vi "hind brain 3.vi"() -> ()   [LabVIEW 2011, in "Hindbrain Demo.lvrbt"]
uses:
  Hindbrain Demo.lvrbt
  <vilib>/NXT/Block Support/HWPage.SensorType.ctl
  <vilib>/NXT/Block Support/HWPage.SensorMode.ctl
  <vilib>/NXT/Block Support/NXT_InputPort.ctl
  <vilib>/NXT/Subs/MotorOutput.ctl
  <vilib>/NXT/HiTechnic/HiTechnic Controls/HiTechnic Port.ctl
  <vilib>/NXT/Dual Mode Library/Motors/MotorBrake.vi
  <vilib>/NXT/Dual Mode Library/Motors/MotorOn.vi
  <vilib>/NXT/Dual Mode Library/Motors/MotorReverse.vi
  New Sensors/mindsensors.com_LVEE_Toolkit/mindsensors.com_LVEE_Toolkit_V1.23/mindsensors.com LVEE Toolkit/Dual/Distance Sensor-DM.vi
  New Sensors/mindsensors.com_LVEE_Toolkit/mindsensors.com_LVEE_Toolkit_V1.23/mindsensors.com LVEE Toolkit/Dual/NXTServo-DM.vi
panel:
  in  "Thrust\nAction":i32
  out "Distance Value":ext
  out "Signal Strength (Array)":u8[](array[numeric])
  out "Direction (0-9)":i16
  in  "Input of NXTServo 2":T1={"Servo Number"=2, "Position"=1500, "Speed"=0} {"Speed" step=1 scale=0.0..255.0; "Position" min=500 max=2500 step=1 scale=500.0..2500.0; "Servo Number" min=1 max=8 step=1}
  out "Output of NXTServo 2":cluster{"Voltage":u8, "Status":bool}
  in  "stop":bool
  in  "Input of NXTServo":T1={"Servo Number"=1, "Position"=1500, "Speed"=0} {"Speed" step=1 scale=0.0..255.0; "Position" min=500 max=2500 step=1 scale=500.0..2500.0; "Servo Number" min=1 max=8 step=1}
  out "Output of NXTServo":cluster{"Voltage":u8, "Status":bool}
  out "Blink":bool
  out "Battery mv":i32
  out "Scaled Value":i16
  out "Left?":bool
  out "Right?":bool
  out "Front?":bool
  out "Stuff?":bool
  # "This is a demonstration of how to sense and acturate devices on the LEGO NXT brick.\nThe connections to the NXT brick are as follows:\nA LEGO gear head motor is connecgted to Port A\nNOTHING IS CONNECTED TO PORTS B AND C.\nPort 1 has the Mindsensor NXTServo\nPort 2 has the HI Technic Infared Seeker\nPort 3 has the Mindsensor DIST - Nx-V3 IR distance sensor\nPort 4 and the Mindsensor NXTSumoEyes-v3."
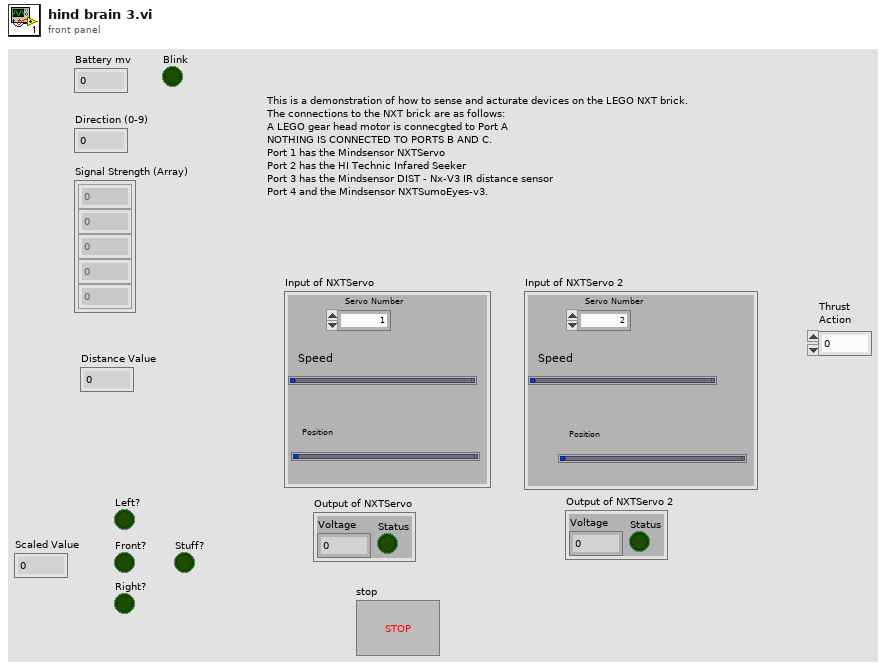
[diagram p1: front panel]
types:
  T1 = cluster{"Servo Number":u8, "Position":u16, "Speed":u8}
  T2 = typedef "MotorOutput.ctl" = u8
  T3 = typedef "NXT_InputPort.ctl" = u8
  T4 = typedef "HWPage.SensorType.ctl" = u8
  T5 = typedef "HWPage.SensorMode.ctl" = u8
  T6 = typedef "LVHSConnector.ctl" = cluster{"Hardware":string, "Flattened String":string}
  T7 = typedef "HiTechnic Port.ctl" = cluster{"Port":T3, "MUX Port":u8}
  T8 = cluster{"Direction (0-9)":i16, "Signal Strength (Array)":u8[]}
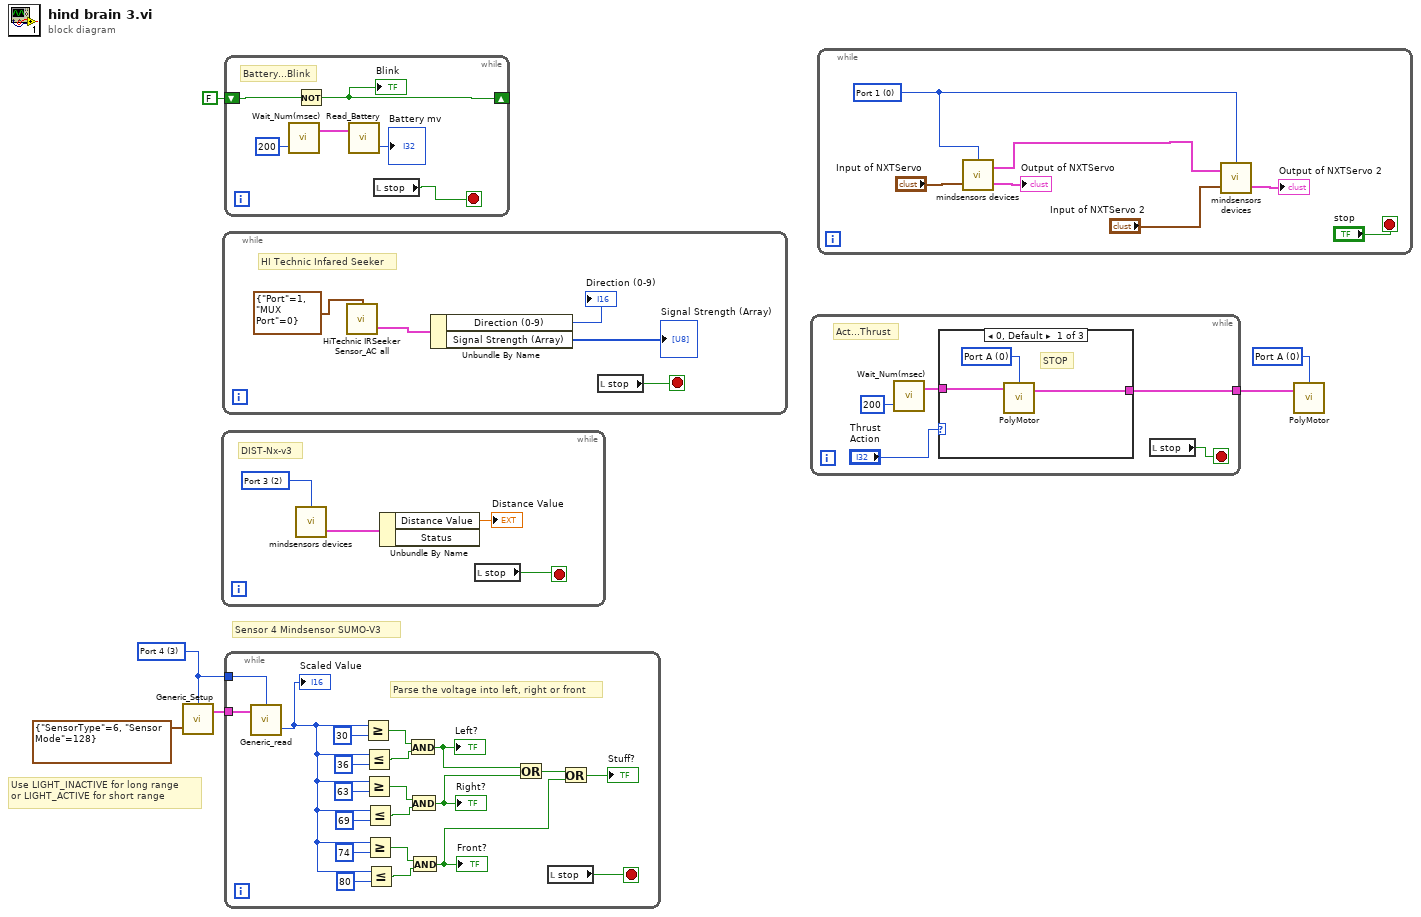
[diagram p0: block diagram]
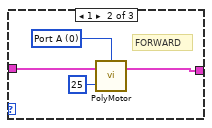
[diagram p2: hidden frame]
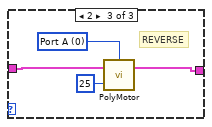
[diagram p3: hidden frame]
diagram:
  w1 = T2 0 items=["Port A"=0, "Port B"=1, "Port C"=2, "Ports A & B"=4, "Ports A & C"=5, "Ports B & C"=6, "All Ports"=3] ("Port (All Ports)")
  w3 = T3 3 items=["Port 1", "Port 2", "Port 3", "Port 4"] ("Port")
  # "Sensor 4 Mindsensor SUMO-V3"
  # "Use LIGHT_INACTIVE for long range\nor LIGHT_ACTIVE for short range"
  n1 = call <vilib>:"Generic_Setup.vi"("Sensor Setup"=cluster{"SensorType":T4, "Sensor Mode":T5} {"SensorType"=6, "Sensor Mode"=128}, "Port"=w3) -> ("NXT"=w6:T6)  [unwired: 1 in, 1 out]
  n2 = while {
    stop <- w10 stop-if-true
    w8 = T3 2 items=["Port 1", "Port 2", "Port 3", "Port 4"] ("Input Port")
    # "DIST-Nx-v3"
    n3 = call-poly "mindsensors devices.vi"("Input Port"=w8) -> ("Output of Distance Sensor"=w9:cluster{"Distance Value":ext, "Status":bool})  [unwired: 2 in, 1 out]
    n4 = Unbundle By Name(w9) -> ("Distance Value"=→"Distance Value":ext)  [unwired: 1 out]
    n5 = local read "stop"() -> (w10:bool)
  }
  n6 = while {
    stop <- w15 stop-if-true
    # "HI Technic Infared Seeker"
    n7 = call <vilib>:"HiTechnic IRSeeker Sensor_AC all.vi"("Port/MUX"=T7 {"Port"=1, "MUX Port"=0}) -> ("All Info"=w13:T8)  [unwired: 2 in, 1 out]
    n8 = Unbundle By Name(w13) -> ("Direction (0-9)"=→"Direction (0-9)":i16, "Signal Strength (Array)"=→"Signal Strength (Array)":u8[])
    n9 = local read "stop"() -> (w15:bool)
  }
  n10 = while {
    shift-right: [w17] -> _
    shift-left: FALSE -> [w18]
    stop <- w19 stop-if-true
    # "Battery...Blink"
    n11 = call <vilib>:"Wait_Num(msec).vi"("Time (100 msec)"=u32 200) -> ("NXT"=w20:T6)  [unwired: 3 in]
    n12 = Not(x=w18) -> (.not. x?=w17:bool)
    "Blink" <- w17
    n13 = call <vilib>:"Read_Battery.vi"("NXT"=w20) -> ("millivolts"=→"Battery mv":i32)  [unwired: 2 in, 1 out]
    n14 = local read "stop"() -> (w19:bool)
  }
  n15 = while {
    tunnel: w3 -> [w42]
    tunnel: w6 -> [w41]
    stop <- w22 stop-if-true
    # "Parse the voltage into left, right or front"
    n16 = call <vilib>:"Generic_read.vi"("NXT"=w41, "Port (Port 3)"=w42) -> ("Scaled Value"=w28:i16)  [unwired: 2 out]
    "Scaled Value" <- w28
    n17 = Greater Or Equal?(x=w28, y=i16 30) -> (x >= y?=w38:bool)
    n18 = Less Or Equal?(x=w28, y=i16 36) -> (x <= y?=w37:bool)
    n19 = Greater Or Equal?(x=w28, y=i16 63) -> (x >= y?=w35:bool)
    n20 = Less Or Equal?(x=w28, y=i16 69) -> (x <= y?=w36:bool)
    n21 = Greater Or Equal?(x=w28, y=i16 74) -> (x >= y?=w31:bool)
    n22 = Less Or Equal?(x=w28, y=i16 80) -> (x <= y?=w32:bool)
    n23 = And(x=w38, y=w37) -> (x .and. y?=w27:bool)
    "Left?" <- w27
    n24 = And(x=w35, y=w36) -> (x .and. y?=w26:bool)
    "Right?" <- w26
    n25 = And(x=w31, y=w32) -> (x .and. y?=w24:bool)
    "Front?" <- w24
    n26 = Or(x=w27, y=w26) -> (x .or. y?=w25:bool)
    n27 = local read "stop"() -> (w22:bool)
    n28 = Or(x=w25, y=w24) -> (x .or. y?=→"Stuff?":bool)
  }
  n29 = while {
    tunnel: [w44] -> w2
    stop <- w46 stop-if-true
    # "Act...Thrust"
    n30 = call <vilib>:"Wait_Num(msec).vi"("Time (100 msec)"=u32 200) -> ("NXT"=w45:T6)  [unwired: 3 in]
    n31 = case shown="0, Default" "Thrust\nAction" {
      tunnel: w45 -> [w50 w54 w58]
      tunnel: [w48 w52 w56] -> w44
      frame 0, Default {
        w49 = T2 0 items=["Port A"=0, "Port B"=1, "Port C"=2, "Ports A & B"=4, "Ports A & C"=5, "Ports B & C"=6, "All Ports"=3] ("Port (All Ports)")
        # "STOP"
        n32 = call-poly <vilib>:"PolyMotor.vi"("NXT"=w50, "Port (All Ports)"=w49) -> ("NXT"=w48:T6)  [unwired: 2 in]
      }
      frame 1 {
        w53 = T2 0 items=["Port A"=0, "Port B"=1, "Port C"=2, "Ports A & B"=4, "Ports A & C"=5, "Ports B & C"=6, "All Ports"=3] ("Output Port (All Ports)")
        # "FORWARD"
        n33 = call-poly <vilib>:"PolyMotor.vi"("Power (75)"=25, "NXT"=w54, "Output Port (All Ports)"=w53) -> ("NXT"=w52:T6)  [unwired: 1 in]
      }
      frame 2 {
        w57 = T2 0 items=["Port A"=0, "Port B"=1, "Port C"=2, "Ports A & B"=4, "Ports A & C"=5, "Ports B & C"=6, "All Ports"=3] ("Output Port (All Ports)")
        # "REVERSE"
        n34 = call-poly <vilib>:"PolyMotor.vi"("Power (75)"=25, "NXT"=w58, "Output Port (All Ports)"=w57) -> ("NXT"=w56:T6)  [unwired: 1 in]
      }
    }
    n35 = local read "stop"() -> (w46:bool)
  }
  n36 = while {
    stop <- "stop" stop-if-true
    w59 = T3 0 items=["Port 1", "Port 2", "Port 3", "Port 4"] ("Input Port")
    n37 = call-poly "mindsensors devices.vi"("Input of NXTServo"="Input of NXTServo", "Input Port"=w59) -> ("Output of NXTServo"=→"Output of NXTServo":cluster{"Voltage":u8, "Status":bool}, "NXT dup"=w60:T6)  [unwired: 1 in]
    n38 = call-poly "mindsensors devices.vi"("Input of NXTServo"="Input of NXTServo 2", "NXT"=w60, "Input Port"=w59) -> ("Output of NXTServo"=→"Output of NXTServo 2":cluster{"Voltage":u8, "Status":bool})  [unwired: 1 out]
  }
  n39 = call-poly <vilib>:"PolyMotor.vi"("NXT"=w2, "Port (All Ports)"=w1) -> ()  [unwired: 2 in, 1 out]
